vi "InitHH_UIThread.vi"(8 "error in (no error)":errorcluster, 9 "mode":T2 items=["Histo"=0, "T2"=2, "T3"=3, "Conti"=8], 10 "refsource":T3, 11 "Library Version":string="3.0") -> (0 "error out":errorcluster, 2 "Init Info":T1, 3 "DevIdx":i32)   [LabVIEW 2010]
uses:
  HH_InitInfo.ctl
  HH_MeasMode.ctl
  HH_RefSource.ctl
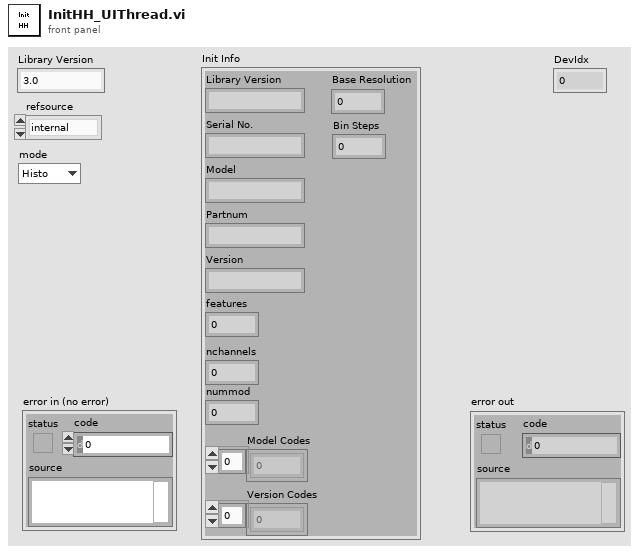
[diagram p1: front panel]
types:
  T1 = typedef "HH_InitInfo.ctl" = cluster{"Library Version":string, "Serial No.":string, "Model":string, "Partnum":string, "Version":string, "features":i32, "nchannels":i32, "nummod":i32, "Model Codes":i32[], "Version Codes":i32[], "Base Resolution":dbl, "Bin Steps":i32}
  T2 = typedef "HH_MeasMode.ctl" = i32
  T3 = typedef "HH_RefSource.ctl" = enum16{"internal", "external"}
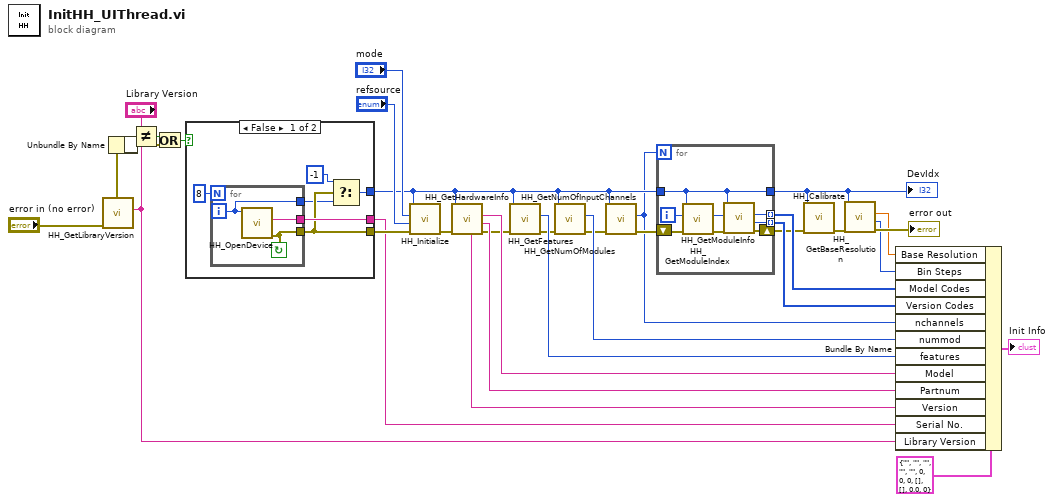
[diagram p0: block diagram]
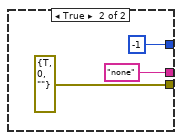
[diagram p2: hidden frame]
diagram:
  n1 = call "HH_GetLibraryVersion.vi"("error in (no error)"="error in (no error)") -> ("error out"=w32:errorcluster, "Version"=w19:string)  [unwired: 8 in, 1 out]
  n2 = Not Equal?(x="Library Version", y=w19) -> (x != y?=w31:bool)
  n3 = Or(x=w31) -> (y=w1:errorcluster, x .or. y?=w30:bool)
  n4 = Unbundle By Name(w32, w1) -> ()
  n5 = case shown="False" w30 {
    tunnel: [w35 -1 ("return type")] -> w12
    tunnel: [w38 "none" ("serial")] -> w21
    tunnel: [w37 errorcluster {"status"=TRUE, "code"=0, "source"=""} ("error out")] -> w29
    frame False {
      n6 = for {
        N: 8 -> [_]
        tunnel: [w41] -> w37
        tunnel: [w40] -> w38
        tunnel: [w42] -> w36
        i -> [w42]
        stop <- w41 continue-if-true
        n7 = call "HH_OpenDevice.vi"("devidx"=w42) -> ("error out"=w41:errorcluster, "serial"=w40:string)  [unwired: 8 in, 1 out]
      }
      n8 = Select(t=-1, s=w37, f=w36) -> (s? t:f=w35:i32)
    }
    frame True {
    }
  }
  n9 = call "HH_Initialize.vi"("error in (no error)"=w29, "refsource"="refsource", "mode"="mode", "devidx"=w12) -> ("error out"=w26:errorcluster)  [unwired: 6 in, 1 out]
  n10 = call "HH_GetHardwareInfo.vi"("error in (no error)"=w26, "devidx"=w12) -> ("error out"=w17:errorcluster, "Partnum"=w24:string, "Model"=w25:string, "Version"=w23:string)  [unwired: 5 in, 1 out]
  n11 = call "HH_GetFeatures.vi"("error in (no error)"=w17, "devidx"=w12) -> ("error out"=w16:errorcluster, "features"=w22:i32)  [unwired: 7 in, 1 out]
  n12 = call "HH_GetNumOfModules.vi"("error in (no error)"=w16, "devidx"=w12) -> ("error out"=w14:errorcluster, "nummod"=w15:i32)  [unwired: 7 in, 1 out]
  n13 = call "HH_GetNumOfInputChannels.vi"("error in (no error)"=w14, "devidx"=w12) -> ("error out"=w13:errorcluster, "nchannels"=w11:i32)  [unwired: 7 in, 1 out]
  n14 = for {
    N: w11 -> [_]
    tunnel: w12 -> [w47]
    tunnel: [w50] -> w10 mode=indexing
    tunnel: [w49] -> w9 mode=indexing
    tunnel: [w47] -> w6
    shift-right: [w46] -> w8
    shift-left: w13 -> [w53]
    i -> [w48]
    n15 = call "HH_GetModuleIndex.vi"("error in (no error)"=w53, "channel"=w48, "devidx"=w47) -> ("error out"=w51:errorcluster, "modidx"=w52:i32)  [unwired: 6 in, 1 out]
    n16 = call "HH_GetModuleInfo.vi"("error in (no error)"=w51, "modidx"=w52, "devidx"=w47) -> ("error out"=w46:errorcluster, "versioncode"=w50:i32, "modelcode"=w49:i32)  [unwired: 5 in, 1 out]
  }
  "DevIdx" <- w6
  n17 = call "HH_Calibrate.vi"("error in (no error)"=w8, "devidx"=w6) -> ("error out"=w7:errorcluster)  [unwired: 8 in, 1 out]
  n18 = call "HH_GetBaseResolution.vi"("error in (no error)"=w7, "devidx"=w6) -> ("error out"=→"error out":errorcluster, "binsteps"=w4:i32, "resolution"=w3:dbl)  [unwired: 6 in, 1 out]
  n19 = Bundle By Name(cluster=T1 {"Library Version"="", "Serial No."="", "Model"="", "Partnum"="", "Version"="", "features"=0, "nchannels"=0, "nummod"=0, "Model Codes"=[], "Version Codes"=[], "Base Resolution"=0.0, "Bin Steps"=0} ("Init"), "Base Resolution"=w3, "Bin Steps"=w4, "Model Codes"=w9, "Version Codes"=w10, "nchannels"=w11, "nummod"=w15, "features"=w22, "Model"=w25, "Partnum"=w24, "Version"=w23, "Serial No."=w21, "Library Version"=w19) -> (→"Init Info":T1)
